vi "7280 Invalid Field--error.vi"(8 "error in":errorcluster, 11 "field":string) -> (0 "error out":errorcluster)   [LabVIEW 2024, in "SourceGrid.lvlib"]
uses:
  SourceGrid.lvlib
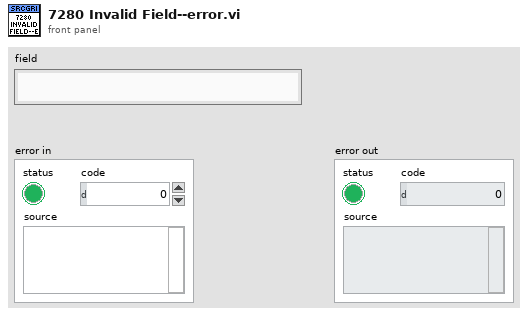
[diagram p1: front panel]
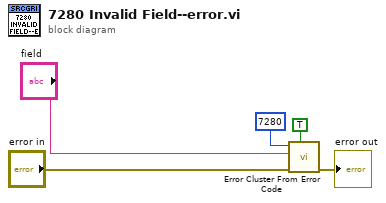
[diagram p0: block diagram]
diagram:
  n1 = call <vilib>:"Error Cluster From Error Code.vi"("show call chain? (False)"=TRUE, "error in (no error)"="error in", "error message (\"\")"="field", "error code (0)"=7280) -> ("error out"=→"error out":errorcluster)  [unwired: 5 in]
